vi "Update.vi"(8 "error in":errorcluster, 11 "CRD Subject in":refnum<class "CRD Subject.lvclass">) -> (0 "error out":errorcluster, 2 "Stop?":bool, 3 "CRD Subject out":refnum<class "CRD Subject.lvclass">)   [LabVIEW 2015, in "CRD Subject.lvclass"]
doc: "Data for the photoacoustic is retrieved via a shared variable 'Data'. The Update VI checks the SV for fresh data. If there is fresh data, then the 'Data' string is unflattened to the proper type (in this case cCRDS Data), stuffed into the DVR (the 'Preserve Runtime Class' VI is required to handle the cast in the 'In Place Element Structure') and the observers are notified via a new element in the queue."
uses:
  CRD Subject.lvclass
  Reusable/Data/Data.lvclass
  Reusable/CRDS/Data/Main/CRDS Data.lvclass
  Reusable/Observer/Data Subject.lvclass/Data Subject.ctl
  Reusable/Observer/Accessors/Read Observer Refs.vi
  Reusable/Observer/Accessors/Read DVR.vi
  Reusable/Observer/Data Subject.lvclass
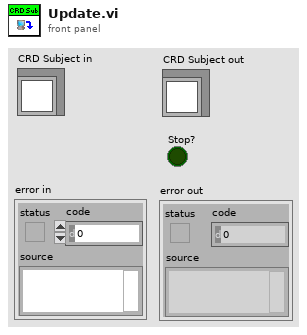
[diagram p1: front panel]
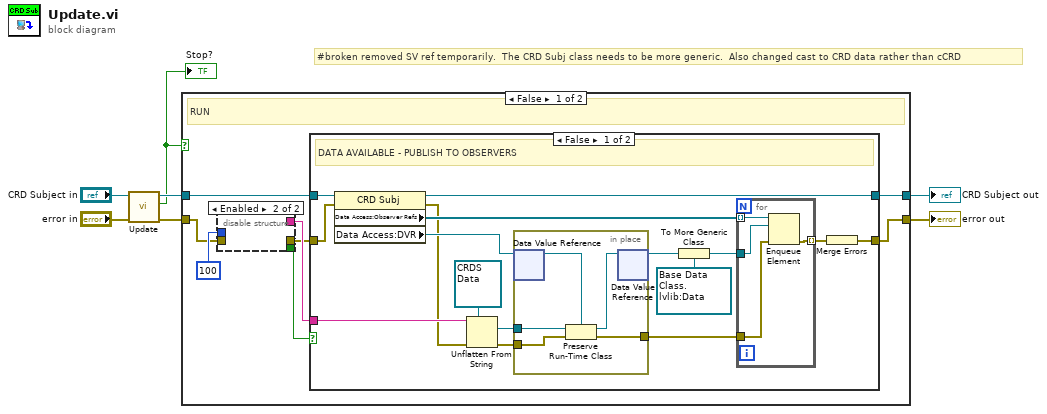
[diagram p0: block diagram]
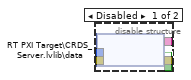
[diagram p2: hidden frame]
diagram:
  # "#broken removed SV ref temporarily.  The CRD Subj class needs to be more generic.  Also changed cast to CRD data rather than cCRD"
  n1 = call-parent "Update.vi"("error in"="error in", "Data Subject in"="CRD Subject in") -> ("error out"=w3:errorcluster, "Stop?"=w4:bool, "Data Subject out"=w5:refnum<class "CRD Subject.lvclass">)  [unwired: 7 in]
  "Stop?" <- w4
  n2 = case shown="False" w4 {
    tunnel: w5 -> [w12 w49]
    tunnel: [w11 w49] -> w2
    tunnel: [w9 w48] -> w1
    tunnel: w3 -> [w8 w48]
    frame False {
      # "RUN"
      n3 = disable-structure shown="Enabled" {
        disable-tunnel: 100 ("ms timeout (0)") -> [w20 _]
        disable-tunnel: [w19 _] -> w14
        disable-tunnel: [w18 _] -> w13
        disable-tunnel: [w17 _] -> w10
        disable-tunnel: w8 -> [w16 _]
        frame Disabled {
          n4 = shared-variable "RT PXI Target\\CRDS_Server.lvlib\\data"(error in=w16, w20) -> (w19:string, error out=w17:errorcluster, w18:bool)
        }
        frame Enabled {
        }
      }
      n5 = case shown="False" w13 {
        tunnel: w14 -> [w33 _]
        tunnel: w12 -> [w32 w47]
        tunnel: [w29 w47] -> w11
        tunnel: w10 -> [w28 w46]
        tunnel: [w22 w46] -> w9
        frame False {
          # "DATA AVAILABLE - PUBLISH TO OBSERVERS"
          n6 = property class="CRD Subj"(reference=w32, error in=w28) -> (reference out=w29:refnum<class "CRD Subject.lvclass">, error out=w23:errorcluster, "Data Access:Observer Refs"=w31:refnum<queue>[], "Data Access:DVR"=w30:refnum<data-value>)
          n7 = Unflatten From String(type=refnum<class "CRDS Data.lvclass"> refnum ("CRDS"), binary string=w33, error in (no error)=w23) -> (value=w34:refnum<class "CRDS Data.lvclass">, error out=w25:errorcluster)  [unwired: 2 in, 1 out]
          n8 = in-place {
            in-place-border: w34 -> [w45]
            in-place-border: [w42] -> w24
            in-place-border: w25 -> [w41]
            n9 = in-place-dvr #1(w30) -> (w44:refnum<class "Data.lvclass">)  [unwired: 1 out]
            n10 = Preserve Run-Time Class(object in=w45, error in=w41, 2:w44) -> (object out=w43:refnum<class "Data.lvclass">, error out=w42:errorcluster)
            n11 = in-place-dvr #1(w43) -> (w36:refnum<data-value>)  [unwired: 1 out]
          }
          n12 = To More Generic Class(target class=refnum<data-value> refnum ("data value reference"), reference=w36) -> (generic class reference=w35:refnum<data-value>)
          n13 = for {
            tunnel: w35 -> [w40]
            tunnel: w31 -> [w39] mode=indexing
            tunnel: w24 -> [w38]
            tunnel: [w37] -> w21 mode=indexing
            n14 = Enqueue Element(queue=w39, element=w40, error in (no error)=w38) -> (error out=w37:errorcluster)  [unwired: 1 in, 2 out]
          }
          n15 = Merge Errors(w21) -> (w22:errorcluster)
        }
        frame True {
          # "NO DATA AVAILABLE"
        }
      }
    }
    frame True {
      # "STOP"
    }
  }
  "error out" <- w1
  "CRD Subject out" <- w2
